vi "Teleop.vi"(10 "Match Info":T1={"Autonomous Elapsed Seconds"=0.0, "TeleOp Elapsed Seconds"=0.0, "Disabled Elapsed Seconds"=0.0, "Visited Autonomous"=FALSE, "Visited TeleOp"=FALSE, "Visited Disabled"=FALSE, "Autonomous Settings"={"Autonomous Style"=enum."Independent", "VI Refnum"=refnum}}, 11 "Call Context":T2) -> ()   [LabVIEW 2013]
doc: "This VI is called for each TeleOp packet received from the DS where the robot is not disabled. It is often used to read from the joysticks and update I/O or to update setpoints for timed control loops. It should complete and return within 20 milliseconds or it may miss DS packets."
uses:
  <vilib>/Rock Robotics/WPI/DriverStation/WPI_DriverStationDerivedRobotMode.ctl
  <vilib>/Rock Robotics/WPI/DriverStation/WPI_DriverStationMatch Info.ctl
  <vilib>/Rock Robotics/WPI/Solenoid/WPI_SolenoidValue.ctl
  Robot Global Data.vi
  <vilib>/Rock Robotics/WPI/Solenoid/Deprecated/WPI_SolenoidGetBool.vi
  <vilib>/Rock Robotics/WPI/Solenoid/WPI_SolenoidSetEnum.vi
  POT.vi
  Voltage.vi
  <vilib>/Rock Robotics/WPI/Joystick/WPI_JoystickGetSetRefNum.vi
  <vilib>/Rock Robotics/WPI/RobotDrive/WPI_RobotDriveGetSetRefNum.vi
panel:
  out "Voltage":dbl
  out "POT Value  2":dbl
  out "POT Value 3":dbl
  out "POT Value":dbl
  out "Numeric 1":dbl(slide) scale=0.0..100.0
  out "Boolean 2":bool
  out "Boolean 1":bool
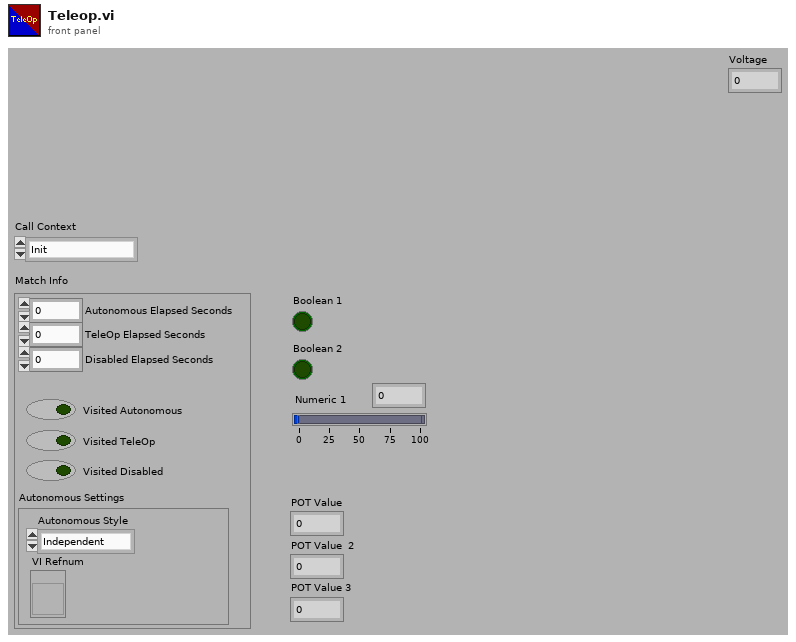
[diagram p1: front panel]
types:
  T1 = typedef "WPI_DriverStationMatch Info.ctl" = cluster{"Autonomous Elapsed Seconds":dbl, "TeleOp Elapsed Seconds":dbl, "Disabled Elapsed Seconds":dbl, "Visited Autonomous":bool, "Visited TeleOp":bool, "Visited Disabled":bool, "Autonomous Settings":cluster{"Autonomous Style":enum16{"Iterative", "Independent"}, "VI Refnum":refnum<vi>}}
  T2 = typedef "WPI_DriverStationDerivedRobotMode.ctl" = enum16{"Init", "Execute", "Stop"}
  T3 = typedef "WPI_JoystickDevRef.ctl" = cluster{"Device":T4}
  T4 = typedef "WPI_JoystickDeviceEnum.ctl" = enum16{"USB 1", "USB 2", "USB 3", "USB 4", "Kinect 1", "Kinect 2"}
  T5 = typedef "WPI_JoystickButtonState.ctl" = cluster{"Button 1":bool, "Button 2":bool, "Button 3":bool, "Button 4":bool, "Button 5":bool, "Button 6":bool, "Button 7":bool, "Button 8":bool, "Button 9":bool, "Button 10":bool, "Button 11":bool, "Button 12":bool}
  T6 = typedef "WPI_RobotDriveDevRef.ctl" = cluster{"DevStatus":errorcluster, "Motors[]":T7[], "Square Inputs":bool, "Max Output":dbl, "Isochronous":bool}
  T7 = typedef "WPI_MotorControlDeviceRef.ctl" = cluster{"DeviceStatus":errorcluster, "Type":enum16{"PWM", "CAN"}, "PWM":cluster{"Digital Module":T8, "PWM Channel":T9, "DeadBand":T10}, "CAN":cluster{"Device Number":u8, "Control Mode":T11, "Semaphore":T12, "Max Vout":dbl}, "Invert":bool, "TransformRef":T13, "InvTransformRef":T13}
  T8 = typedef "FPGA_TypedefDigitalModule.ctl" = enum16{"Digital Module 1", "Digital Module 2"}
  T9 = typedef "FPGA_DIOPWMChannel.ctl" = enum8{"PWM 1", "PWM 2", "PWM 3", "PWM 4", "PWM 5", "PWM 6", "PWM 7", "PWM 8", "PWM 9", "PWM 10", "Invalid"}
  T10 = typedef "WPI_PWMDeadband.ctl" = cluster{"Name":string, "maxPositivePwm":i32, "minPositivePwm":i32, "centerPwm":i32, "maxNegativePwm":i32, "minNegativePwm":i32, "angularRange":u16}
  T11 = typedef "WPI_CANJaguar_ControlMode.ctl" = enum8{"Percent VBus", "Current", "Speed", "Position", "Voltage"}
  T12 = typedef "Semaphore RefNum" = refnum<k1>
  T13 = typedef "WPI_PWMTransform_ConPane.ctl" = refnum<vi>
  T14 = cluster{"axis 1 (x)":dbl, "axis 2 (y)":dbl, "axis 3 (throttle)":dbl, "axis 4":dbl, "axis 5":dbl, "axis 6":dbl}
  T15 = typedef "WPI_SolenoidDevRef.ctl" = cluster{"DevStatus":errorcluster, "Solenoid Module":T16, "Forward Solenoid Channel":T17, "Reverse Solenoid Channel":T17}
  T16 = typedef "FPGA_TypedefSolenoidModule.ctl" = enum16{"Solenoid Module 1", "Solenoid Module 2"}
  T17 = typedef "WPI_SolenoidChannel.ctl" = enum8{"Solenoid 1", "Solenoid 2", "Solenoid 3", "Solenoid 4", "Solenoid 5", "Solenoid 6", "Solenoid 7", "Solenoid 8", "Invalid"}
  T18 = typedef "WPI_SolenoidValue.ctl" = enum16{"Off", "On", "Forward", "Reverse"}
  T19 = typedef "WPI_RelayDevRef.ctl" = cluster{"DevStatus":errorcluster, "Relay Channel":T20, "Digital Module":T8, "Relay Direction":T21}
  T20 = typedef "FPGA_DIORelayChannel.ctl" = enum8{"Relay 1", "Relay 2", "Relay 3", "Relay 4", "Relay 5", "Relay 6", "Relay 7", "Relay 8", "Invalid"}
  T21 = typedef "WPI_RelayDirection.ctl" = enum16{"Both directions", "Forward only", "Reverse only"}
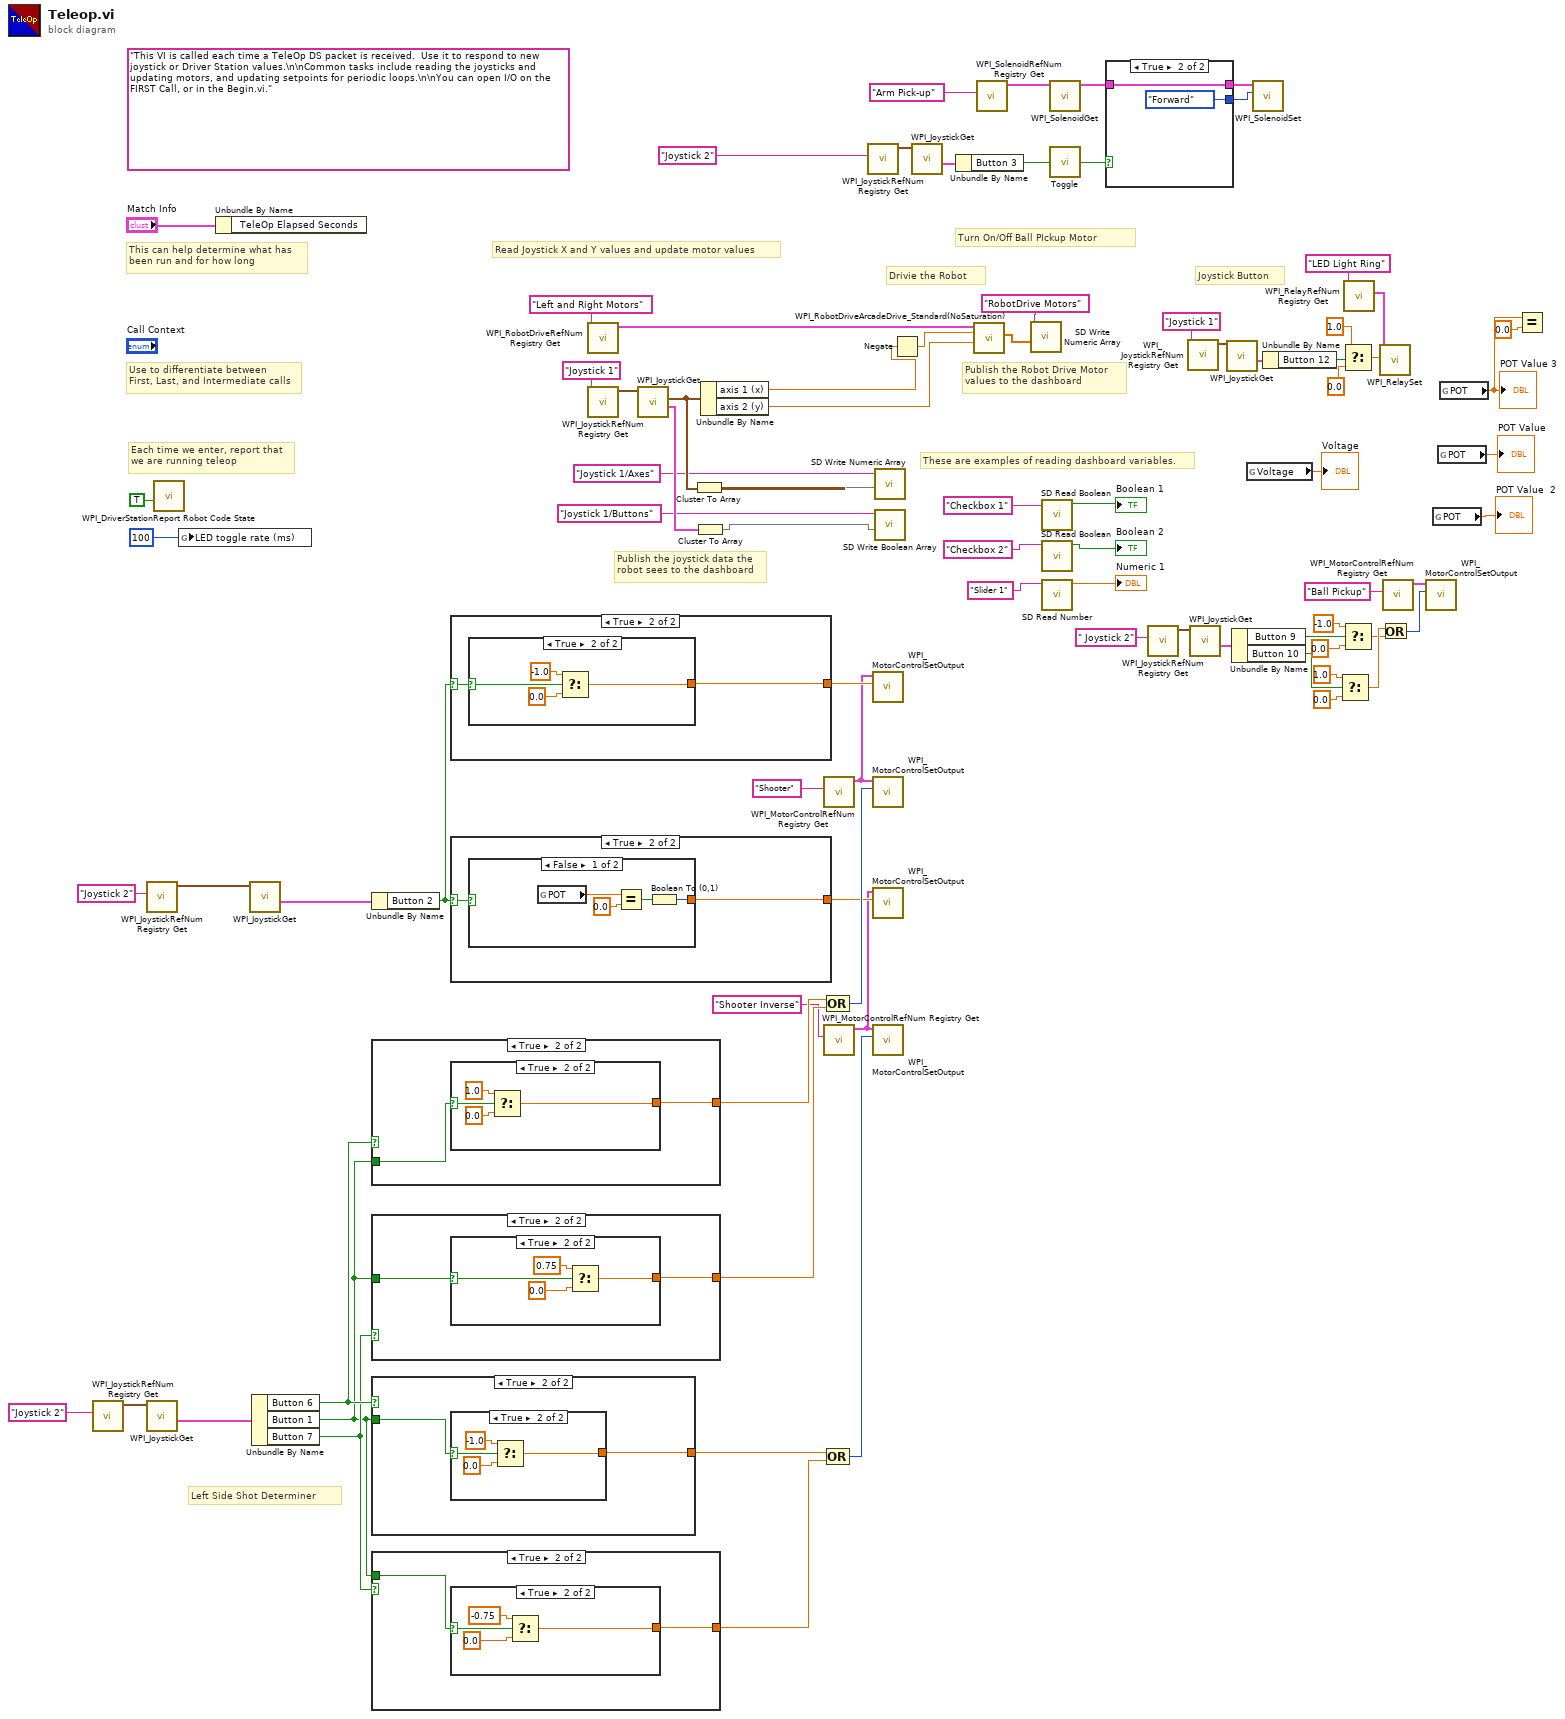
[diagram p0: block diagram]
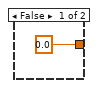
[diagram p2: hidden frame]
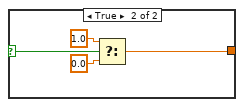
[diagram p3: hidden frame]
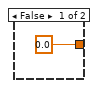
[diagram p4: hidden frame]
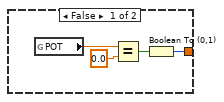
[diagram p5: hidden frame]
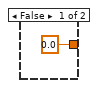
[diagram p6: hidden frame]
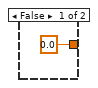
[diagram p7: hidden frame]
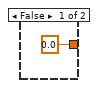
[diagram p8: hidden frame]
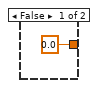
[diagram p9: hidden frame]
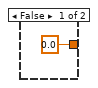
[diagram p10: hidden frame]
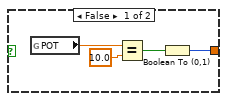
[diagram p11: hidden frame]
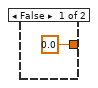
[diagram p12: hidden frame]
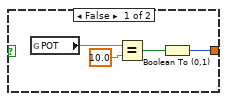
[diagram p13: hidden frame]
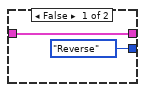
[diagram p14: hidden frame]
diagram:
  (unwired) "This VI is called each time a TeleOp DS packet is received.  Use it to respond to new joystick or Driver Station values.\n\nCommon tasks include reading the joysticks and updating motors, and updating setpoints for periodic loops.\n\nYou can open I/O on the FIRST Call, or in the Begin.vi."
  # "Left Side Shot Determiner"
  # "Turn On/Off Ball PIckup Motor"
  # "Joystick Button"
  # "Drivie the Robot"
  # "These are examples of reading dashboard variables."
  # "Publish the Robot Drive Motor\nvalues to the dashboard"
  # "Publish the joystick data the\nrobot sees to the dashboard"
  # "Each time we enter, report that\nwe are running teleop"
  # "Use to differentiate between\nFirst, Last, and Intermediate calls"
  # "This can help determine what has\nbeen run and for how long"
  # "Read Joystick X and Y values and update motor values"
  n1 = call <vilib>:"WPI_JoystickRefNum Registry Get.vi"("refnum name"="Joystick 2") -> ("JoystickDevRef"=w15:T3)  [unwired: 9 in, 1 out]
  n2 = call <vilib>:"WPI_JoystickRefNum Registry Get.vi"("refnum name"="Joystick 2") -> ("JoystickDevRef"=w10:T3)  [unwired: 9 in, 1 out]
  n3 = call <vilib>:"WPI_JoystickGet.vi"("JoystickDevRef"=w15) -> ("Buttons"=w16:T5)  [unwired: 4 in, 2 out]
  n4 = call <vilib>:"WPI_DriverStationReport Robot Code State.vi"("TeleOp"=TRUE ("Autonomous")) -> ()  [unwired: 10 in, 1 out]
  n5 = global write "Robot Global Data.vi" "LED toggle rate (ms)"(u32 100 ("LED ms toggle rate")) -> ()
  n6 = Unbundle By Name("Match Info") -> ()  [unwired: 1 out]
  n7 = call <vilib>:"WPI_JoystickGet.vi"("JoystickDevRef"=w10) -> ("Buttons"=w9:T5)  [unwired: 4 in, 2 out]
  n8 = Unbundle By Name(w16) -> ("Button 6"=w3:bool, "Button 1"=w1:bool, "Button 7"=w2:bool)
  n9 = Unbundle By Name(w9) -> ("Button 2"=w8:bool)
  n10 = case shown="True" w3 {
    tunnel: [0.0 ("f") w87] -> w20
    tunnel: w1 -> [_ w86]
    frame False {
    }
    frame True {
      n11 = case shown="True" w86 {
        selector: w86 -> [_ w93]
        tunnel: [w88 w92] -> w87
        frame False {
          n12 = global read "POT.vi" "POT"() -> (w91:dbl)
          n13 = Equal?(x=w91, y=10.0) -> (x = y?=w89:bool)
          n14 = Boolean To (0,1)(Boolean=w89) -> (0, 1=w88:i16)
        }
        frame True {
          n15 = Select(t=1.0, s=w93, f=0.0) -> (s? t:f=w92:dbl)
        }
      }
    }
  }
  n16 = case shown="True" w2 {
    tunnel: [0.0 ("f") w98] -> w21
    tunnel: w1 -> [_ w97]
    frame False {
    }
    frame True {
      n17 = case shown="True" w97 {
        selector: w97 -> [_ w104]
        tunnel: [w99 w103] -> w98
        frame False {
          n18 = global read "POT.vi" "POT"() -> (w100:dbl)
          n19 = Equal?(x=w100, y=10.0) -> (x = y?=w102:bool)
          n20 = Boolean To (0,1)(Boolean=w102) -> (0, 1=w99:i16)
        }
        frame True {
          n21 = Select(t=0.75, s=w104, f=0.0) -> (s? t:f=w103:dbl)
        }
      }
    }
  }
  n22 = case shown="True" w3 {
    tunnel: w1 -> [_ w109]
    tunnel: [0.0 ("f") w108] -> w17
    frame False {
    }
    frame True {
      n23 = case shown="True" w109 {
        selector: w109 -> [_ w112]
        tunnel: [0.0 ("f") w111] -> w108
        frame False {
        }
        frame True {
          n24 = Select(t=-1.0, s=w112, f=0.0) -> (s? t:f=w111:dbl)
        }
      }
    }
  }
  n25 = case shown="True" w2 {
    tunnel: w1 -> [_ w117]
    tunnel: [0.0 ("f") w116] -> w18
    frame False {
    }
    frame True {
      n26 = case shown="True" w117 {
        selector: w117 -> [_ w120]
        tunnel: [0.0 ("f") w119] -> w116
        frame False {
        }
        frame True {
          n27 = Select(t=-0.75, s=w120, f=0.0) -> (s? t:f=w119:dbl)
        }
      }
    }
  }
  n28 = case shown="True" w8 {
    selector: w8 -> [_ w124]
    tunnel: [0.0 ("f") w125] -> w6
    frame False {
    }
    frame True {
      n29 = case shown="True" w124 {
        selector: w124 -> [_ w131]
        tunnel: [w126 w130] -> w125
        frame False {
          n30 = global read "POT.vi" "POT"() -> (w128:dbl)
          n31 = Equal?(x=w128, y=0.0) -> (x = y?=w127:bool)
          n32 = Boolean To (0,1)(Boolean=w127) -> (0, 1=w126:i16)
        }
        frame True {
          n33 = Select(t=-1.0, s=w131, f=0.0) -> (s? t:f=w130:dbl)
        }
      }
    }
  }
  n34 = case shown="True" w8 {
    selector: w8 -> [_ w135]
    tunnel: [0.0 ("f") w136] -> w7
    frame False {
    }
    frame True {
      n35 = case shown="False" w135 {
        selector: w135 -> [_ w144]
        tunnel: [w137 w141] -> w136
        frame False {
          n36 = global read "POT.vi" "POT"() -> (w140:dbl)
          n37 = Equal?(x=w140, y=0.0) -> (x = y?=w138:bool)
          n38 = Boolean To (0,1)(Boolean=w138) -> (0, 1=w137:i16)
        }
        frame True {
          n39 = Select(t=1.0, s=w144, f=0.0) -> (s? t:f=w141:dbl)
        }
      }
    }
  }
  n40 = call <vilib>:"WPI_RobotDriveRefNum Registry Get.vi"("refnum name"="Left and Right Motors") -> ("RobotDriveDevRef"=w82:T6)  [unwired: 1 in, 9 out]
  n41 = call <vilib>:"WPI_JoystickRefNum Registry Get.vi"("refnum name"="Joystick 1") -> ("JoystickDevRef"=w79:T3)  [unwired: 1 in, 9 out]
  n42 = call <vilib>:"WPI_JoystickGet.vi"("JoystickDevRef"=w79) -> ("Buttons"=w76:T5, "Axes"=w73:T14)  [unwired: 1 in, 4 out]
  n43 = Cluster To Array(cluster=w73) -> (array=w72:dbl[])
  n44 = Cluster To Array(cluster=w76) -> (array=w75:bool[])
  n45 = Unbundle By Name(w73) -> ("axis 1 (x)"=w47:dbl, "axis 2 (y)"=w81:dbl)
  n46 = call <vilib>:"WPI_MotorControlRefNum Registry Get.vi"("refnum name"="Shooter") -> ("MotorControlDevRef"=w5:T7)  [unwired: 9 in, 1 out]
  n47 = call <vilib>:"WPI_MotorControlRefNum Registry Get.vi"("refnum name"="Shooter Inverse") -> ("MotorControlDevRef"=w4:T7)  [unwired: 9 in, 1 out]
  n48 = Compound Arithmetic op=OR(w20, w21) -> (w22:i32)
  n49 = Compound Arithmetic op=OR(w17, w18) -> (w19:i32)
  n50 = call <vilib>:"WPI_JoystickRefNum Registry Get.vi"("refnum name"="Joystick 2") -> ("JoystickDevRef"=w49:T3)  [unwired: 9 in, 1 out]
  n51 = call <vilib>:"WPI_MotorControlSetOutput.vi"("Output"=w6, "MotorControlDevRef"=w5) -> ()  [unwired: 7 in, 3 out]
  n52 = call <vilib>:"WPI_MotorControlSetOutput.vi"("Output"=w22, "MotorControlDevRef"=w5) -> ()  [unwired: 7 in, 3 out]
  n53 = call <vilib>:"WPI_MotorControlSetOutput.vi"("Output"=w7, "MotorControlDevRef"=w4) -> ()  [unwired: 7 in, 3 out]
  n54 = call <vilib>:"WPI_MotorControlSetOutput.vi"("Output"=w19, "MotorControlDevRef"=w4) -> ()  [unwired: 7 in, 3 out]
  n55 = call <vilib>:"SD Write Numeric Array.vi"("Numeric Array"=w72, "Name"="Joystick 1/Axes") -> ()  [unwired: 8 in, 2 out]
  n56 = call <vilib>:"SD Write Boolean Array.vi"("Boolean Array"=w75, "Name"="Joystick 1/Buttons") -> ()  [unwired: 8 in, 2 out]
  n57 = Negate(x=w47) -> (-x=w46:dbl)
  n58 = call <vilib>:"WPI_JoystickGet.vi"("JoystickDevRef"=w49) -> ("Buttons"=w48:T5)  [unwired: 4 in, 2 out]
  n59 = Unbundle By Name(w48) -> ("Button 3"=w45:bool)
  n60 = call <vilib>:"WPI_RobotDriveArcadeDrive_Standard(NoSaturation).vi"("Y axis value"=w81, "X axis value"=w46, "RobotDriveDevRef"=w82) -> ("Motor Values"=w69:dbl[])  [unwired: 1 in, 7 out]
  n61 = call <vilib>:"WPI_SolenoidRefNum Registry Get.vi"("refnum name"="Arm Pick-up") -> ("SolenoidDevRef"=w32:T15)  [unwired: 9 in, 1 out]
  n62 = call <vilib>:"SD Write Numeric Array.vi"("Numeric Array"=w69, "Name"="RobotDrive Motors") -> ()  [unwired: 8 in, 2 out]
  n63 = call <vilib>:"SD Read Boolean.vi"("Name"="Checkbox 1" ("refnum name")) -> ("Boolean"=→"Boolean 1":bool)  [unwired: 8 in, 2 out]
  n64 = call <vilib>:"SD Read Boolean.vi"("Name"="Checkbox 2" ("refnum name")) -> ("Boolean"=→"Boolean 2":bool)  [unwired: 8 in, 2 out]
  n65 = call <vilib>:"SD Read Number.vi"("Name"="Slider 1" ("refnum name")) -> ("Numeric"=→"Numeric 1":dbl)  [unwired: 8 in, 2 out]
  n66 = call-poly <vilib>:"WPI_SolenoidGet.vi"("SolenoidDevRef"=w32) -> ("SolenoidDevRef"=w30:T15)  [unwired: 8 in, 2 out]
  n67 = call "Toggle.vi"("Input"=w45) -> ("Toggled Output"=w31:bool)
  n68 = case shown="True" w31 {
    tunnel: w30 -> [w146 w148]
    tunnel: [w146 w148] -> w29
    tunnel: [WPI_SolenoidValue."Reverse" ("Value") WPI_SolenoidValue."Forward" ("Value")] -> w28
    frame False {
    }
    frame True {
    }
  }
  n69 = call <vilib>:"WPI_JoystickRefNum Registry Get.vi"("refnum name"=" Joystick 2") -> ("JoystickDevRef"=w38:T3)  [unwired: 9 in, 1 out]
  n70 = call <vilib>:"WPI_JoystickRefNum Registry Get.vi"("refnum name"="Joystick 1") -> ("JoystickDevRef"=w58:T3)  [unwired: 9 in, 1 out]
  n71 = call <vilib>:"WPI_JoystickGet.vi"("JoystickDevRef"=w38) -> ("Buttons"=w39:T5)  [unwired: 4 in, 2 out]
  n72 = call <vilib>:"WPI_JoystickGet.vi"("JoystickDevRef"=w58) -> ("Buttons"=w57:T5)  [unwired: 4 in, 2 out]
  n73 = Unbundle By Name(w39) -> ("Button 9"=w40:bool, "Button 10"=w36:bool)
  n74 = global read "Voltage.vi" "Voltage"() -> (→"Voltage":dbl)
  n75 = call-poly <vilib>:"WPI_SolenoidSet.vi"("Value"=w28, "SolenoidDevRef"=w29) -> ()  [unwired: 8 in, 2 out]
  n76 = Unbundle By Name(w57) -> ("Button 12"=w56:bool)
  n77 = Select(t=1.0, s=w36, f=0.0) -> (s? t:f=w35:dbl)
  n78 = Select(t=1.0, s=w56, f=0.0) -> (s? t:f=w55:dbl)
  n79 = Select(t=-1.0, s=w40, f=0.0) -> (s? t:f=w34:dbl)
  n80 = call <vilib>:"WPI_RelayRefNum Registry Get.vi"("refnum name"="LED Light Ring") -> ("RelayDevRef"=w62:T19)  [unwired: 9 in, 1 out]
  n81 = call <vilib>:"WPI_RelaySet.vi"("RelayValue"=w55, "RelayDevRef"=w62) -> ()  [unwired: 8 in, 2 out]
  n82 = Or(x=w35, y=w34) -> (x .or. y?=w33:i32)
  n83 = call <vilib>:"WPI_MotorControlRefNum Registry Get.vi"("refnum name"="Ball Pickup") -> ("MotorControlDevRef"=w52:T7)  [unwired: 9 in, 1 out]
  n84 = call <vilib>:"WPI_MotorControlSetOutput.vi"("Output"=w33, "MotorControlDevRef"=w52) -> ()  [unwired: 7 in, 3 out]
  n85 = global read "POT.vi" "POT"() -> (→"POT Value  2":dbl)
  n86 = global read "POT.vi" "POT"() -> (→"POT Value":dbl)
  n87 = global read "POT.vi" "POT"() -> (w27:dbl)
  "POT Value 3" <- w27
  n88 = Equal?(x=w27, y=0.0) -> ()  [unwired: 1 out]
